vi "[Global] RootPath.vi"() -> ()   [LabVIEW 2019]
panel:
  out "RootPath":path
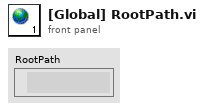
[diagram p1: front panel]
diagram:
